vi "Calculate Resistance Specs.vi"(8 "Tol %":dbl, 11 "Nom Value":dbl) -> (0 "Tol Range":dbl, 1 "Deviation":dbl, 2 "Lower Limit":dbl, 3 "Upper Limit":dbl)   [LabVIEW 2018, in "Resistance Value.lvlib"]
doc: "Calculates the resistor specifications from the nominal resistance value and tolerance.\n\nThe VI receives the <b>Nom Value</b> and <b>Tol %</b> and calculates the corresponding <b>Deviation</b>, <b>Upper Limit</b>, <b>Lower Limit</b>, and <b>Tol Range</b>."
uses:
  Resistance Value/Resistance Value.lvlib
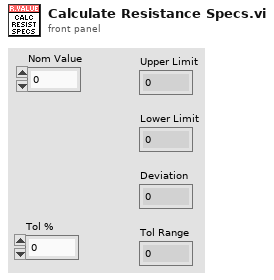
[diagram p1: front panel]
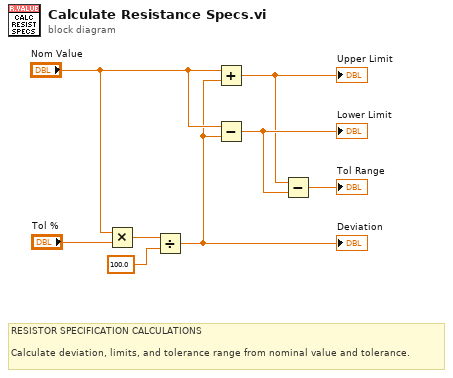
[diagram p0: block diagram]
diagram:
  # "RESISTOR SPECIFICATION CALCULATIONS\n\nCalculate deviation, limits, and tolerance range from nominal value and tolerance."
  n1 = Multiply(x="Nom Value", y="Tol %") -> (x*y=w4:dbl)
  n2 = Divide(x=w4, y=100.0) -> (x/y=w1:dbl)
  "Deviation" <- w1
  n3 = Add(x="Nom Value", y=w1) -> (x+y=w2:dbl)
  "Upper Limit" <- w2
  n4 = Subtract(x="Nom Value", y=w1) -> (x-y=w8:dbl)
  "Lower Limit" <- w8
  n5 = Subtract(x=w2, y=w8) -> (x-y=→"Tol Range":dbl)
